vi "Autonomous Independent.vi"() -> ()   [LabVIEW 2017]
doc: "This VI is called when autonomous begins, and will automatically be terminated when autonomous ends. You can carry out timed or sensor driven robot movement independently without needing to return to the caller."
uses:
  <vilib>/Rock Robotics/WPI/ThirdParty/Sensors/navX/_TypeDefs/FRIC_navX_DeviceNumbersTypeDef.ctl
  <vilib>/Rock Robotics/WPI/Utilities/WPI_GetSetVariantRefNum.vi
  <vilib>/addons/control/pid/pid.llb/PID (DBL).vi
  <vilib>/addons/control/pid/NI_PID_pid.lvlib
  <vilib>/Rock Robotics/WPI/RobotDrive/WPI_RobotDriveArcadeDrive_Standard(NoSaturation).vi
panel:
  out "Angle 2":dbl
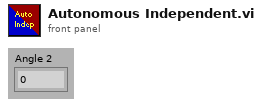
[diagram p1: front panel]
types:
  T1 = typedef "WPI_EncoderDevRef.ctl" = cluster{"DevStatus":errorcluster, "EncoderIndex":T2, "CounterIndex":T3, "DistancePerCount":dbl, "Decoding Type":T4}
  T2 = typedef "FPGA_EncoderIdx.ctl" = enum8{"Enc 0", "Enc 1", "Enc 2", "Enc 3", "Enc 4", "Enc 5", "Enc 6", "Enc 7", "Invalid"}
  T3 = typedef "FPGA_CounterCtrSystemIndex.ctl" = enum8{"Ctr 0", "Ctr 1", "Ctr 2", "Ctr 3", "Ctr 4", "Ctr 5", "Ctr 6", "Ctr 7", "Invalid"}
  T4 = typedef "WPI_EncoderType.ctl" = enum16{"1x", "2x", "4x"}
  T5 = typedef "WPI_RobotDriveDevRef.ctl" = cluster{"DevStatus":errorcluster, "Motors[]":T6[], "Square Inputs":bool, "Max Output":dbl}
  T6 = typedef "WPI_MotorControlDeviceRef.ctl" = cluster{"DeviceStatus":errorcluster, "Type":T7, "PWM":cluster{"PWM Channel":T8, "DeadBand":T9}, "CAN":cluster{"Device Number":u8, "SetOutput VI Ref":variant, "GetOutput VI Ref":variant, "Enable VI Ref":variant, "Disable VI Ref":variant, "Data":variant}, "Invert":bool, "DIO PWM":cluster{"PWM \"Enable\" Channel":T8, "DIOChannel":T10, "PWM Rate":dbl}}
  T7 = typedef "WPI_MotorControlType.ctl" = enum16{"PWM", "CAN", "DIO PWM"}
  T8 = typedef "FPGA_DIOPWMChannel.ctl" = enum8{"PWM 0", "PWM 1", "PWM 2", "PWM 3", "PWM 4", "PWM 5", "PWM 6", "PWM 7", "PWM 8", "PWM 9", "PWM MXP 0", "PWM MXP 1", "PWM MXP 2", "PWM MXP 3", "PWM MXP 4", "PWM MXP 5", "PWM MXP 6", "PWM MXP 7", "PWM MXP 8", "PWM MXP 9", "Invalid"}
  T9 = typedef "WPI_PWMDeadband.ctl" = cluster{"Name":string, "maxPositivePwm":i32, "minPositivePwm":i32, "centerPwm":i32, "maxNegativePwm":i32, "minNegativePwm":i32, "angularRange":u16}
  T10 = typedef "FPGA_DIOChannel.ctl" = enum8{"DIO 0", "DIO 1", "DIO 2", "DIO 3", "DIO 4", "DIO 5", "DIO 6", "DIO 7", "DIO 8", "DIO 9", "DIO MXP 0", "DIO MXP 1", "DIO MXP 2", "DIO MXP 3", "DIO MXP 4", "DIO MXP 5", "DIO MXP 6", "DIO MXP 7", "DIO MXP 8", "DIO MXP 9", "DIO MXP 10", "DIO MXP 11", "DIO MXP 12", "DIO MXP 13", "DIO MXP 14", "DIO MXP 15", "SPI Port CS1", "SPI Port CS2", "SPI Port CS3", "SPI Port MISO", "SPI Port MOSI", "Invalid"}
  T11 = typedef "WPI_GyroDevRef.ctl" = cluster{"DevStatus":errorcluster, "Analog Channel":T12, "Gain (VoltsPerDegree/Second)":dbl, "Gyro Type":enum16{"Analog", "XRS450"}, "Handle":i32, "SPI Bus":T13, "Device Found":bool, "Sample Rate":dbl, "Calibrate On Open":bool, "Offset":dbl}
  T12 = typedef "FPGA_AIChannel.ctl" = enum8{"AI 0", "AI 1", "AI 2", "AI 3", "AI MXP 0", "AI MXP 1", "AI MXP 2", "AI MXP 3", "Invalid"}
  T13 = typedef "spi_bus.ctl" = enum16{"SPI On-Board, CS0", "SPI On-Board, CS1", "SPI On-Board, CS2", "SPI On-Board, CS3", "SPI MXP", "Invalid"}
  T14 = typedef "FRIC_navX_DeviceNumbersTypeDef.ctl" = enum16{"Dev0", "Dev1", "Dev2", "Dev3"}
  T15 = cluster{"proportional gain (Kc)":dbl, "integral time (Ti, min)":dbl, "derivative time (Td, min)":dbl}
  T16 = cluster{"Yaw":dbl, "Roll":dbl, "Pitch":dbl, "Heading":dbl, "Fused Heading":dbl}
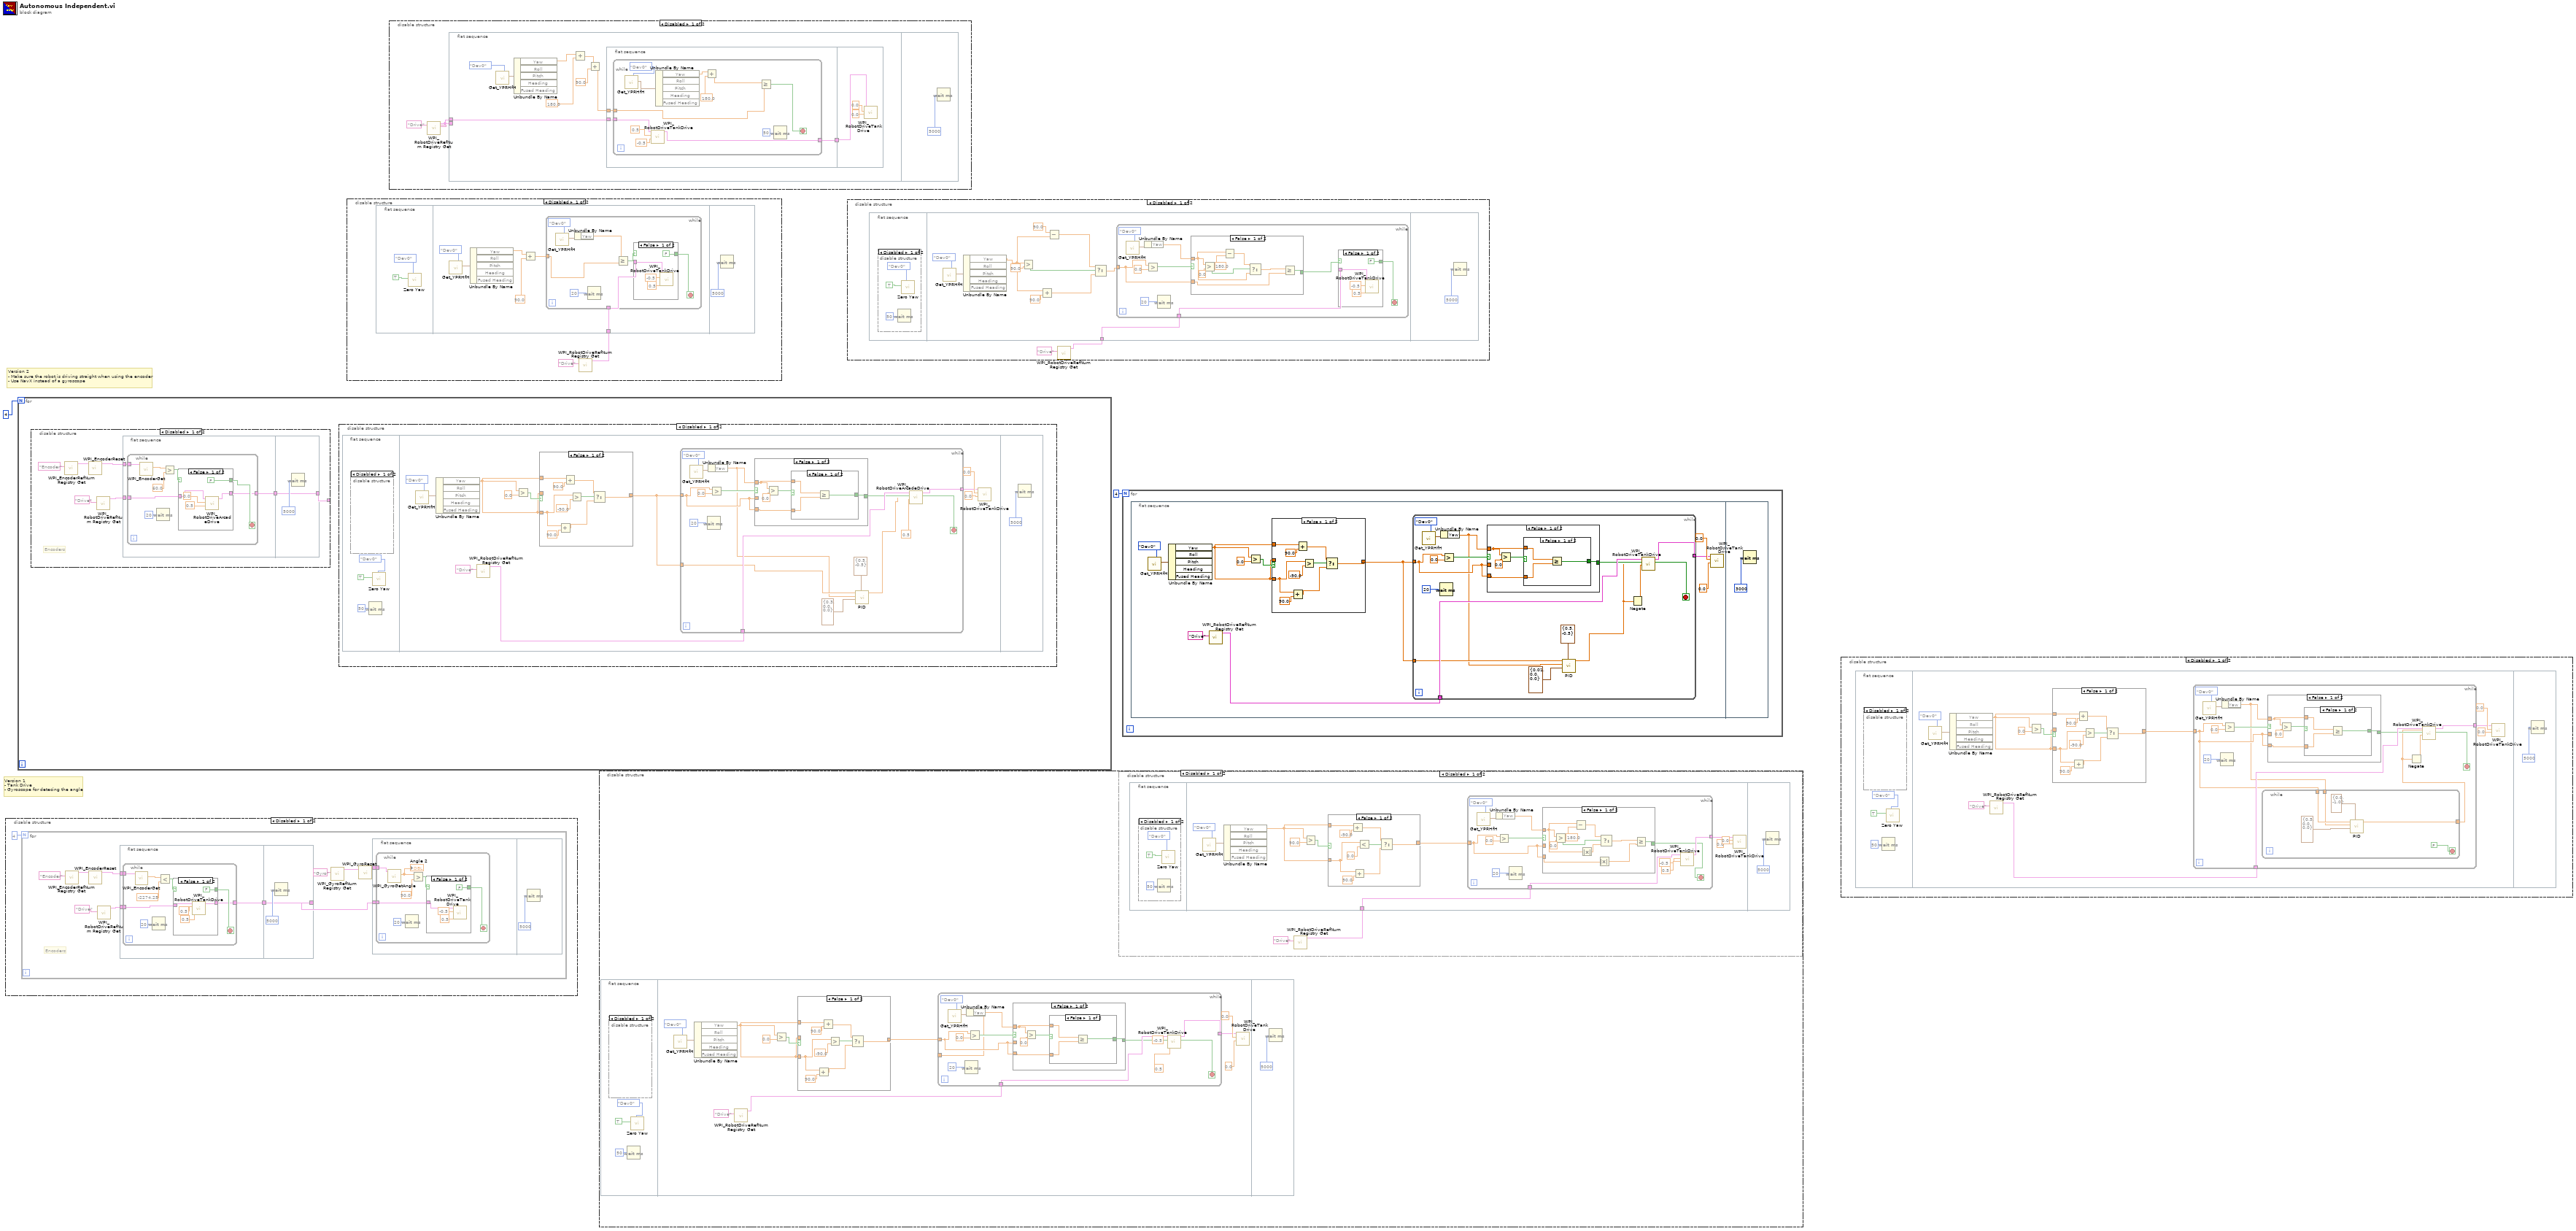
[diagram p0: block diagram]
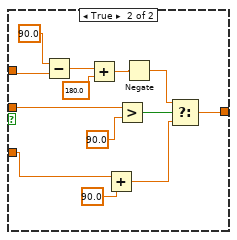
[diagram p2: hidden frame]
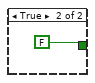
[diagram p3: hidden frame]
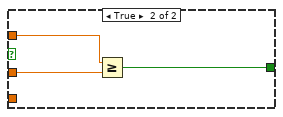
[diagram p4: hidden frame]
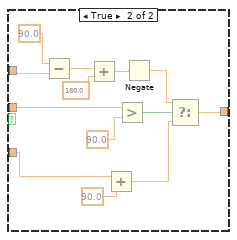
[diagram p6: hidden frame]
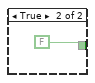
[diagram p7: hidden frame]
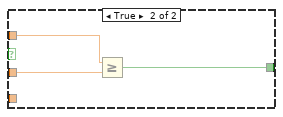
[diagram p8: hidden frame]
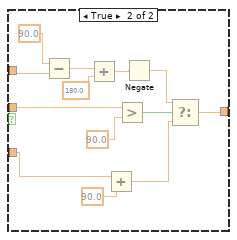
[diagram p11: hidden frame]
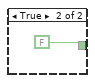
[diagram p12: hidden frame]
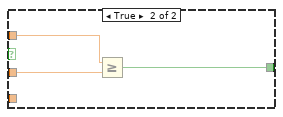
[diagram p13: hidden frame]
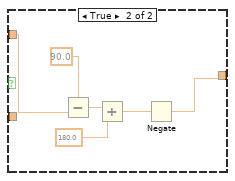
[diagram p15: hidden frame]
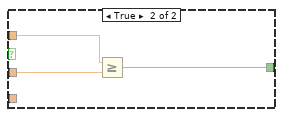
[diagram p16: hidden frame]
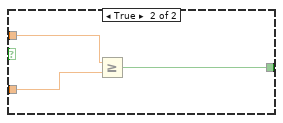
[diagram p20: hidden frame]
diagram:
  # "Version 2\n- Make sure the robot is driving straight when using the encoder\n- Use NavX instead of a gyroscope"
  # "Version 1\n- Tank Drive\n- Gyroscope for detecing the angle"
  n1 = disable-structure shown="Disabled" {
    frame Disabled {
      n2 = for {
        N: 4 -> [_]
        # "Encoders"
        n3 = call <vilib>:"WPI_EncoderRefNum Registry Get.vi"("refnum name"="Encoder") -> ("EncoderDevRef"=w10:T1)  [unwired: 9 in, 1 out]
        n4 = call <vilib>:"WPI_EncoderReset.vi"("EncoderDevRef"=w10) -> ("EncoderDevRef"=w9:T1)  [unwired: 9 in, 1 out]
        n5 = call <vilib>:"WPI_RobotDriveRefNum Registry Get.vi"("refnum name"="Drive") -> ("RobotDriveDevRef"=w13:T5)  [unwired: 9 in, 1 out]
        n6 = flat-sequence {
          tunnel: w9 -> [w34]
          tunnel: w13 -> [w33]
          tunnel: [w32] -> w4
          tunnel: [w53] -> w5
          tunnel: w4 -> [w53]
          frame #0 {
            n7 = while {
              tunnel: w34 -> [w42]
              tunnel: w33 -> [w38]
              tunnel: [w35] -> w32
              stop <- w41 stop-if-true
              n8 = call <vilib>:"WPI_EncoderGet.vi"("EncoderDevRef"=w42) -> ("Distance"=w39:dbl)  [unwired: 5 in, 5 out]
              n9 = Wait (ms)(milliseconds to wait=u32 20) -> ()  [unwired: 1 out]
              n10 = Less?(x=w39, y=-2274.25) -> (x < y?=w40:bool)
              n11 = case shown="False" w40 {
                tunnel: [FALSE TRUE] -> w41
                tunnel: w38 -> [w45 w49]
                tunnel: [w46 w48] -> w35
                frame False {
                  n12 = call <vilib>:"WPI_RobotDriveTankDrive.vi"("Right axis value"=0.5, "Left axis value"=0.5, "RobotDriveDevRef"=w45) -> ("RobotDriveDevRef"=w46:T5)  [unwired: 6 in, 2 out]
                }
                frame True {
                  n13 = call <vilib>:"WPI_RobotDriveTankDrive.vi"("Right axis value"=0.0, "Left axis value"=0.0, "RobotDriveDevRef"=w49) -> ("RobotDriveDevRef"=w48:T5)  [unwired: 6 in, 2 out]
                }
              }
            }
          }
          frame #1 {
            n14 = Wait (ms)(milliseconds to wait=u32 5000) -> ()  [unwired: 1 out]
          }
        }
        n15 = call <vilib>:"WPI_GyroRefNum Registry Get.vi"("refnum name"="Gyro") -> ("GyroDevRef"=w7:T11)  [unwired: 9 in, 1 out]
        n16 = call <vilib>:"WPI_GyroReset.vi"("GyroDevRef"=w7) -> ("GyroDevRef"=w8:T11)  [unwired: 9 in, 1 out]
        n17 = flat-sequence {
          tunnel: w8 -> [w15]
          tunnel: w5 -> [w14]
          frame #0 {
            n18 = while {
              tunnel: w15 -> [w18]
              tunnel: w14 -> [w16]
              stop <- w22 stop-if-true
              n19 = call <vilib>:"WPI_GyroGetAngle.vi"("GyroDevRef"=w18) -> ("Angle"=w17:dbl)  [unwired: 6 in, 4 out]
              "Angle 2" <- w17
              n20 = Wait (ms)(milliseconds to wait=u32 20) -> ()  [unwired: 1 out]
              n21 = Greater?(x=w17, y=90.0) -> (0:w21:bool)
              n22 = case shown="False" w21 {
                tunnel: [FALSE TRUE] -> w22
                tunnel: w16 -> [w23 w27]
                frame False {
                  n23 = call <vilib>:"WPI_RobotDriveTankDrive.vi"("Right axis value"=0.5, "Left axis value"=-0.5, "RobotDriveDevRef"=w23) -> ()  [unwired: 6 in, 3 out]
                }
                frame True {
                  n24 = call <vilib>:"WPI_RobotDriveTankDrive.vi"("Right axis value"=0.0, "Left axis value"=0.0, "RobotDriveDevRef"=w27) -> ()  [unwired: 6 in, 3 out]
                }
              }
            }
          }
          frame #1 {
            n25 = Wait (ms)(milliseconds to wait=u32 5000) -> ()  [unwired: 1 out]
          }
        }
      }
    }
    frame Enabled {
    }
  }
  n26 = for {
    N: 4 -> [_]
    n27 = disable-structure shown="Disabled" {
      disable-tunnel: [w119 _] -> _
      frame Disabled {
        # "Encoders"
        n28 = call <vilib>:"WPI_EncoderRefNum Registry Get.vi"("refnum name"="Encoder") -> ("EncoderDevRef"=w121:T1)  [unwired: 9 in, 1 out]
        n29 = call <vilib>:"WPI_EncoderReset.vi"("EncoderDevRef"=w121) -> ("EncoderDevRef"=w120:T1)  [unwired: 9 in, 1 out]
        n30 = call <vilib>:"WPI_RobotDriveRefNum Registry Get.vi"("refnum name"="Drive") -> ("RobotDriveDevRef"=w124:T5)  [unwired: 9 in, 1 out]
        n31 = flat-sequence {
          tunnel: w120 -> [w128]
          tunnel: w124 -> [w127]
          tunnel: [w126] -> w125
          tunnel: [w147] -> w119
          tunnel: w125 -> [w147]
          frame #0 {
            n32 = while {
              tunnel: w128 -> [w136]
              tunnel: w127 -> [w132]
              tunnel: [w129] -> w126
              stop <- w135 stop-if-true
              n33 = call <vilib>:"WPI_EncoderGet.vi"("EncoderDevRef"=w136) -> ("Distance"=w133:dbl)  [unwired: 5 in, 5 out]
              n34 = Wait (ms)(milliseconds to wait=u32 20) -> ()  [unwired: 1 out]
              n35 = Greater?(x=w133, y=60.0) -> (0:w134:bool)
              n36 = case shown="False" w134 {
                tunnel: [FALSE TRUE] -> w135
                tunnel: w132 -> [w139 w143]
                tunnel: [w140 w142] -> w129
                frame False {
                  n37 = call-poly <vilib>:"WPI_RobotDriveArcadeDrive.vi"("Y axis value"=0.5 ("Right axis value"), "X axis value"=0.0 ("Left axis value"), "RobotDriveDevRef"=w139) -> ("RobotDriveDevRef"=w140:T5)  [unwired: 6 in, 2 out]
                }
                frame True {
                  n38 = call <vilib>:"WPI_RobotDriveTankDrive.vi"("Right axis value"=0.0, "Left axis value"=0.0, "RobotDriveDevRef"=w143) -> ("RobotDriveDevRef"=w142:T5)  [unwired: 6 in, 2 out]
                }
              }
            }
          }
          frame #1 {
            n39 = Wait (ms)(milliseconds to wait=u32 5000) -> ()  [unwired: 1 out]
          }
        }
      }
      frame Enabled {
      }
    }
    n40 = disable-structure shown="Disabled" {
      frame Disabled {
        n41 = flat-sequence {
          frame #0 {
            n42 = disable-structure shown="Disabled" {
              frame Disabled {
              }
              frame Enabled {
              }
            }
            n43 = Wait (ms)(milliseconds to wait=u32 50) -> ()  [unwired: 1 out]
            n44 = call <vilib>:"Zero Yaw.vi"("Device Number"=FRIC_navX_DeviceNumbersTypeDef."Dev0", "Zero"=TRUE) -> ()  [unwired: 10 in]
          }
          frame #1 {
            n45 = call <vilib>:"Get_YPRHfH.vi"("Device Number"=FRIC_navX_DeviceNumbersTypeDef."Dev0") -> ("YRPHfH"=w68:T16)  [unwired: 10 in]
            n46 = Unbundle By Name(w68) -> ("Yaw"=w60:dbl)  [unwired: 4 out]
            n47 = call <vilib>:"WPI_RobotDriveRefNum Registry Get.vi"("refnum name"="Drive") -> ("RobotDriveDevRef"=w59:T5)  [unwired: 9 in, 1 out]
            n48 = Greater?(x=w60, y=0.0) -> (0:w63:bool)
            n49 = case shown="False" w63 {
              tunnel: w60 -> [w74 w82]
              tunnel: w60 -> [w71 w84]
              tunnel: [w72 w87] -> w58
              tunnel: w60 -> [_ w86]
              frame False {
                n50 = Add(x=w71, y=90.0) -> (x+y=w69:dbl)
                n51 = Add(x=w74, y=90.0) -> (x+y=w73:dbl)
                n52 = Greater?(x=w71, y=-90.0) -> (0:w76:bool)
                n53 = Select(t=w73, s=w76, f=w69) -> (s? t:f=w72:dbl)
              }
              frame True {
                n54 = Subtract(x=90.0, y=w82) -> (x-y=w81:dbl)
                n55 = Add(x=w81, y=180.0) -> (x+y=w79:dbl)
                n56 = Add(x=w84, y=90.0) -> (x+y=w88:dbl)
                n57 = Greater?(x=w86, y=90.0) -> (0:w89:bool)
                n58 = Negate(x=w79) -> (-x=w78:dbl)
                n59 = Select(t=w78, s=w89, f=w88) -> (s? t:f=w87:dbl)
              }
            }
            n60 = while {
              tunnel: w59 -> [w102]
              tunnel: [w99] -> w64
              tunnel: w58 -> [w97]
              tunnel: w58 -> [w96]
              stop <- w98 stop-if-true
              n61 = call <vilib>:"Get_YPRHfH.vi"("Device Number"=FRIC_navX_DeviceNumbersTypeDef."Dev0") -> ("YRPHfH"=w104:T16)  [unwired: 10 in]
              n62 = Wait (ms)(milliseconds to wait=u32 20) -> ()  [unwired: 1 out]
              n63 = Unbundle By Name(w104) -> ("Yaw"=w95:dbl)
              n64 = Greater?(x=w97, y=0.0) -> (0:w100:bool)
              n65 = case shown="False" w100 {
                tunnel: w95 -> [w108 w117]
                tunnel: [w106 w116] -> w98
                tunnel: w97 -> [_ w115]
                tunnel: w97 -> [w107 _]
                frame False {
                  n66 = Greater?(x=w108, y=0.0) -> (0:w109:bool)
                  n67 = case shown="False" w109 {
                    tunnel: w108 -> [w113 _]
                    tunnel: w107 -> [w112 _]
                    tunnel: [w111 FALSE] -> w106
                    frame False {
                      n68 = Greater Or Equal?(x=w113, y=w112) -> (x >= y?=w111:bool)
                    }
                    frame True {
                    }
                  }
                }
                frame True {
                  n69 = Greater Or Equal?(x=w117, y=w115) -> (x >= y?=w116:bool)
                }
              }
              n70 = call-poly <vilib>:"PID.vi"("output range"=cluster{"output high":dbl, "output low":dbl} {"output high"=0.5, "output low"=-0.5}, "PID gains"=T15 {"proportional gain (Kc)"=0.3, "integral time (Ti, min)"=0.0, "derivative time (Td, min)"=0.0}, "process variable"=w95, "setpoint"=w96) -> ("output"=w92:dbl)  [unwired: 6 in, 1 out]
              n71 = call-poly <vilib>:"WPI_RobotDriveArcadeDrive.vi"("Y axis value"=0.5, "X axis value"=w92, "RobotDriveDevRef"=w102) -> ("RobotDriveDevRef"=w99:T5)  [unwired: 6 in, 2 out]
            }
            n72 = call <vilib>:"WPI_RobotDriveTankDrive.vi"("Right axis value"=0.0, "Left axis value"=0.0, "RobotDriveDevRef"=w64) -> ()  [unwired: 6 in, 3 out]
          }
          frame #2 {
            n73 = Wait (ms)(milliseconds to wait=u32 5000) -> ()  [unwired: 1 out]
          }
        }
      }
      frame Enabled {
      }
    }
  }
  n74 = disable-structure shown="Disabled" {
    frame Disabled {
      n75 = flat-sequence {
        tunnel: w150 -> [w153]
        frame #0 {
          n76 = call <vilib>:"Zero Yaw.vi"("Device Number"=FRIC_navX_DeviceNumbersTypeDef."Dev0", "Zero"=TRUE) -> ()  [unwired: 10 in]
        }
        frame #1 {
          n77 = call <vilib>:"Get_YPRHfH.vi"("Device Number"=FRIC_navX_DeviceNumbersTypeDef."Dev0") -> ("YRPHfH"=w158:T16)  [unwired: 10 in]
          n78 = Unbundle By Name(w158) -> ("Yaw"=w156:dbl)  [unwired: 4 out]
          n79 = Add(x=w156, y=90.0) -> (x+y=w155:dbl)
          n80 = while {
            tunnel: w155 -> [w163]
            tunnel: w153 -> [w160]
            stop <- w166 stop-if-true
            n81 = call <vilib>:"Get_YPRHfH.vi"("Device Number"=FRIC_navX_DeviceNumbersTypeDef."Dev0") -> ("YRPHfH"=w162:T16)  [unwired: 10 in]
            n82 = Unbundle By Name(w162) -> ("Yaw"=w159:dbl)
            n83 = Wait (ms)(milliseconds to wait=u32 20) -> ()  [unwired: 1 out]
            n84 = Greater Or Equal?(x=w159, y=w163) -> (x >= y?=w165:bool)
            n85 = case shown="False" w165 {
              tunnel: [FALSE TRUE] -> w166
              tunnel: w160 -> [w167 w171]
              frame False {
                n86 = call <vilib>:"WPI_RobotDriveTankDrive.vi"("Right axis value"=0.5, "Left axis value"=-0.5, "RobotDriveDevRef"=w167) -> ()  [unwired: 6 in, 3 out]
              }
              frame True {
                n87 = call <vilib>:"WPI_RobotDriveTankDrive.vi"("Right axis value"=0.0, "Left axis value"=0.0, "RobotDriveDevRef"=w171) -> ()  [unwired: 6 in, 3 out]
              }
            }
          }
        }
        frame #2 {
          n88 = Wait (ms)(milliseconds to wait=u32 5000) -> ()  [unwired: 1 out]
        }
      }
      n89 = call <vilib>:"WPI_RobotDriveRefNum Registry Get.vi"("refnum name"="Drive") -> ("RobotDriveDevRef"=w150:T5)  [unwired: 9 in, 1 out]
    }
    frame Enabled {
    }
  }
  n90 = disable-structure shown="Disabled" {
    frame Disabled {
      n91 = call <vilib>:"WPI_RobotDriveRefNum Registry Get.vi"("refnum name"="Drive") -> ("RobotDriveDevRef"=w177:T5)  [unwired: 9 in, 1 out]
      n92 = flat-sequence {
        tunnel: w177 -> [_]
        tunnel: w177 -> [w182]
        frame #0 {
          n93 = call <vilib>:"Get_YPRHfH.vi"("Device Number"=FRIC_navX_DeviceNumbersTypeDef."Dev0") -> ("YRPHfH"=w186:T16)  [unwired: 10 in]
          n94 = Unbundle By Name(w186) -> ("Yaw"=w179:dbl)  [unwired: 4 out]
          n95 = Add(x=w179, y=180.0) -> (x+y=w180:dbl)
          n96 = Add(x=w180, y=90.0) -> (x+y=w185:dbl)
          n97 = flat-sequence {
            tunnel: w185 -> [w189]
            tunnel: [w188] -> w183
            tunnel: w182 -> [w187]
            tunnel: w183 -> [w202]
            frame #0 {
              n98 = while {
                tunnel: w189 -> [w199]
                tunnel: [w195] -> w188
                tunnel: w187 -> [w196]
                stop <- w198 stop-if-true
                n99 = call <vilib>:"Get_YPRHfH.vi"("Device Number"=FRIC_navX_DeviceNumbersTypeDef."Dev0") -> ("YRPHfH"=w200:T16)  [unwired: 10 in]
                n100 = call <vilib>:"WPI_RobotDriveTankDrive.vi"("Right axis value"=-0.5, "Left axis value"=0.5, "RobotDriveDevRef"=w196) -> ("RobotDriveDevRef"=w195:T5)  [unwired: 6 in, 2 out]
                n101 = Unbundle By Name(w200) -> ("Yaw"=w192:dbl)  [unwired: 4 out]
                n102 = Add(x=w192, y=180.0) -> (x+y=w190:dbl)
                n103 = Greater Or Equal?(x=w190, y=w199) -> (x >= y?=w198:bool)
                n104 = Wait (ms)(milliseconds to wait=u32 50) -> ()  [unwired: 1 out]
              }
            }
            frame #1 {
              n105 = call <vilib>:"WPI_RobotDriveTankDrive.vi"("Right axis value"=0.0, "Left axis value"=0.0, "RobotDriveDevRef"=w202) -> ()  [unwired: 6 in, 3 out]
            }
          }
        }
        frame #1 {
          n106 = Wait (ms)(milliseconds to wait=u32 5000) -> ()  [unwired: 1 out]
        }
      }
    }
    frame Enabled {
    }
  }
  n107 = disable-structure shown="Disabled" {
    frame Disabled {
      n108 = flat-sequence {
        frame #0 {
          n109 = disable-structure shown="Disabled" {
            frame Disabled {
            }
            frame Enabled {
            }
          }
          n110 = Wait (ms)(milliseconds to wait=u32 50) -> ()  [unwired: 1 out]
          n111 = call <vilib>:"Zero Yaw.vi"("Device Number"=FRIC_navX_DeviceNumbersTypeDef."Dev0", "Zero"=TRUE) -> ()  [unwired: 10 in]
        }
        frame #1 {
          n112 = call <vilib>:"Get_YPRHfH.vi"("Device Number"=FRIC_navX_DeviceNumbersTypeDef."Dev0") -> ("YRPHfH"=w219:T16)  [unwired: 10 in]
          n113 = Unbundle By Name(w219) -> ("Yaw"=w209:dbl)  [unwired: 4 out]
          n114 = call <vilib>:"WPI_RobotDriveRefNum Registry Get.vi"("refnum name"="Drive") -> ("RobotDriveDevRef"=w210:T5)  [unwired: 9 in, 1 out]
          n115 = Greater?(x=w209, y=0.0) -> (0:w214:bool)
          n116 = case shown="False" w214 {
            tunnel: w209 -> [w225 w233]
            tunnel: w209 -> [w222 w235]
            tunnel: [w223 w238] -> w212
            tunnel: w209 -> [_ w237]
            frame False {
              n117 = Add(x=w222, y=90.0) -> (x+y=w220:dbl)
              n118 = Add(x=w225, y=90.0) -> (x+y=w224:dbl)
              n119 = Greater?(x=w222, y=-90.0) -> (0:w227:bool)
              n120 = Select(t=w224, s=w227, f=w220) -> (s? t:f=w223:dbl)
            }
            frame True {
              n121 = Subtract(x=90.0, y=w233) -> (x-y=w232:dbl)
              n122 = Add(x=w232, y=180.0) -> (x+y=w230:dbl)
              n123 = Add(x=w235, y=90.0) -> (x+y=w239:dbl)
              n124 = Greater?(x=w237, y=90.0) -> (0:w240:bool)
              n125 = Negate(x=w230) -> (-x=w229:dbl)
              n126 = Select(t=w229, s=w240, f=w239) -> (s? t:f=w238:dbl)
            }
          }
          n127 = while {
            tunnel: w210 -> [w250]
            tunnel: [w246] -> w215
            tunnel: w212 -> [w245]
            tunnel: [w243] -> _
            stop <- w244 stop-if-true
            n128 = call <vilib>:"Get_YPRHfH.vi"("Device Number"=FRIC_navX_DeviceNumbersTypeDef."Dev0") -> ("YRPHfH"=w252:T16)  [unwired: 10 in]
            n129 = Wait (ms)(milliseconds to wait=u32 20) -> ()  [unwired: 1 out]
            n130 = Unbundle By Name(w252) -> ("Yaw"=w243:dbl)
            n131 = Greater?(x=w245, y=0.0) -> (0:w248:bool)
            n132 = case shown="False" w248 {
              tunnel: w243 -> [w256 w265]
              tunnel: [w254 w264] -> w244
              tunnel: w245 -> [_ w263]
              tunnel: w245 -> [w255 _]
              frame False {
                n133 = Greater?(x=w256, y=0.0) -> (0:w257:bool)
                n134 = case shown="False" w257 {
                  tunnel: w256 -> [w261 _]
                  tunnel: w255 -> [w260 _]
                  tunnel: [w259 FALSE] -> w254
                  frame False {
                    n135 = Greater Or Equal?(x=w261, y=w260) -> (x >= y?=w259:bool)
                  }
                  frame True {
                  }
                }
              }
              frame True {
                n136 = Greater Or Equal?(x=w265, y=w263) -> (x >= y?=w264:bool)
              }
            }
            n137 = call <vilib>:"WPI_RobotDriveTankDrive.vi"("Right axis value"=0.5, "Left axis value"=-0.5, "RobotDriveDevRef"=w250) -> ("RobotDriveDevRef"=w246:T5)  [unwired: 6 in, 2 out]
          }
          n138 = call <vilib>:"WPI_RobotDriveTankDrive.vi"("Right axis value"=0.0, "Left axis value"=0.0, "RobotDriveDevRef"=w215) -> ()  [unwired: 6 in, 3 out]
        }
        frame #2 {
          n139 = Wait (ms)(milliseconds to wait=u32 5000) -> ()  [unwired: 1 out]
        }
      }
      n140 = disable-structure shown="Disabled" {
        frame Disabled {
          n141 = flat-sequence {
            tunnel: w268 -> [w279]
            frame #0 {
              n142 = disable-structure shown="Disabled" {
                frame Disabled {
                  n143 = Wait (ms)(milliseconds to wait=u32 50) -> ()  [unwired: 1 out]
                  n144 = call <vilib>:"Zero Yaw.vi"("Device Number"=FRIC_navX_DeviceNumbersTypeDef."Dev0", "Zero"=TRUE) -> ()  [unwired: 10 in]
                }
                frame Enabled {
                }
              }
            }
            frame #1 {
              n145 = call <vilib>:"Get_YPRHfH.vi"("Device Number"=FRIC_navX_DeviceNumbersTypeDef."Dev0") -> ("YRPHfH"=w281:T16)  [unwired: 10 in]
              n146 = Unbundle By Name(w281) -> ("Yaw"=w273:dbl)  [unwired: 4 out]
              n147 = Greater?(x=w273, y=90.0) -> (0:w275:bool)
              n148 = case shown="False" w275 {
                tunnel: w273 -> [w287 w295]
                tunnel: w273 -> [w283 _]
                tunnel: [w282 w291] -> w272
                frame False {
                  n149 = Add(x=w287, y=-90.0) -> (x+y=w285:dbl)
                  n150 = Add(x=w283, y=90.0) -> (x+y=w284:dbl)
                  n151 = Less?(x=w283, y=0.0) -> (x < y?=w289:bool)
                  n152 = Select(t=w285, s=w289, f=w284) -> (s? t:f=w282:dbl)
                }
                frame True {
                  n153 = Subtract(x=90.0, y=w295) -> (x-y=w294:dbl)
                  n154 = Add(x=w294, y=180.0) -> (x+y=w292:dbl)
                  n155 = Negate(x=w292) -> (-x=w291:dbl)
                }
              }
              n156 = while {
                tunnel: w279 -> [w305]
                tunnel: [w299] -> w276
                tunnel: w272 -> [w297]
                stop <- w298 stop-if-true
                n157 = call <vilib>:"Get_YPRHfH.vi"("Device Number"=FRIC_navX_DeviceNumbersTypeDef."Dev0") -> ("YRPHfH"=w307:T16)  [unwired: 10 in]
                n158 = Unbundle By Name(w307) -> ("Yaw"=w302:dbl)
                n159 = Greater?(x=w297, y=0.0) -> (0:w303:bool)
                n160 = Wait (ms)(milliseconds to wait=u32 20) -> ()  [unwired: 1 out]
                n161 = case shown="False" w303 {
                  tunnel: w302 -> [w309 w321]
                  tunnel: [w316 w320] -> w298
                  tunnel: w297 -> [_ w319]
                  tunnel: w297 -> [w312 _]
                  frame False {
                    n162 = Greater?(x=w309, y=0.0) -> (0:w317:bool)
                    n163 = Subtract(x=w309, y=180.0) -> (x-y=w315:dbl)
                    n164 = Absolute Value(x=w309) -> (abs(x)=w310:dbl)
                    n165 = Absolute Value(x=w312) -> (abs(x)=w311:dbl)
                    n166 = Select(t=w315, s=w317, f=w310) -> (s? t:f=w314:dbl)
                    n167 = Greater Or Equal?(x=w314, y=w311) -> (x >= y?=w316:bool)
                  }
                  frame True {
                    n168 = Greater Or Equal?(x=w321, y=w319) -> (x >= y?=w320:bool)
                  }
                }
                n169 = call <vilib>:"WPI_RobotDriveTankDrive.vi"("Right axis value"=0.5, "Left axis value"=-0.5, "RobotDriveDevRef"=w305) -> ("RobotDriveDevRef"=w299:T5)  [unwired: 6 in, 2 out]
              }
              n170 = call <vilib>:"WPI_RobotDriveTankDrive.vi"("Right axis value"=0.0, "Left axis value"=0.0, "RobotDriveDevRef"=w276) -> ()  [unwired: 6 in, 3 out]
            }
            frame #2 {
              n171 = Wait (ms)(milliseconds to wait=u32 5000) -> ()  [unwired: 1 out]
            }
          }
          n172 = call <vilib>:"WPI_RobotDriveRefNum Registry Get.vi"("refnum name"="Drive") -> ("RobotDriveDevRef"=w268:T5)  [unwired: 9 in, 1 out]
        }
        frame Enabled {
        }
      }
    }
    frame Enabled {
    }
  }
  n173 = disable-structure shown="Disabled" {
    frame Disabled {
      n174 = flat-sequence {
        tunnel: w323 -> [w336]
        frame #0 {
          n175 = disable-structure shown="Disabled" {
            frame Disabled {
              n176 = Wait (ms)(milliseconds to wait=u32 50) -> ()  [unwired: 1 out]
              n177 = call <vilib>:"Zero Yaw.vi"("Device Number"=FRIC_navX_DeviceNumbersTypeDef."Dev0", "Zero"=TRUE) -> ()  [unwired: 10 in]
            }
            frame Enabled {
            }
          }
        }
        frame #1 {
          n178 = call <vilib>:"Get_YPRHfH.vi"("Device Number"=FRIC_navX_DeviceNumbersTypeDef."Dev0") -> ("YRPHfH"=w338:T16)  [unwired: 10 in]
          n179 = Unbundle By Name(w338) -> ("Yaw"=w331:dbl)  [unwired: 4 out]
          n180 = Greater?(x=w331, y=90.0) -> (0:w334:bool)
          n181 = Add(x=w331, y=90.0) -> (x+y=w328:dbl)
          n182 = Subtract(x=90.0, y=w331) -> (x-y=w329:dbl)
          n183 = Select(t=w329, s=w334, f=w328) -> (s? t:f=w333:dbl)
          n184 = while {
            tunnel: w336 -> [w344]
            tunnel: w333 -> [w341]
            stop <- w348 stop-if-true
            n185 = call <vilib>:"Get_YPRHfH.vi"("Device Number"=FRIC_navX_DeviceNumbersTypeDef."Dev0") -> ("YRPHfH"=w346:T16)  [unwired: 10 in]
            n186 = Unbundle By Name(w346) -> ("Yaw"=w340:dbl)
            n187 = Greater?(x=w341, y=0.0) -> (0:w342:bool)
            n188 = Wait (ms)(milliseconds to wait=u32 20) -> ()  [unwired: 1 out]
            n189 = case shown="False" w342 {
              tunnel: w341 -> [w354 w359]
              tunnel: w340 -> [w349 w358]
              tunnel: [w353 w357] -> w339
              frame False {
                n190 = Greater?(x=w349, y=0.0) -> (0:w355:bool)
                n191 = Subtract(x=w349, y=180.0) -> (x-y=w352:dbl)
                n192 = Select(t=w352, s=w355, f=w349) -> (s? t:f=w351:dbl)
                n193 = Greater Or Equal?(x=w351, y=w354) -> (x >= y?=w353:bool)
              }
              frame True {
                n194 = Greater Or Equal?(x=w358, y=w359) -> (x >= y?=w357:bool)
              }
            }
            n195 = case shown="False" w339 {
              tunnel: [FALSE TRUE] -> w348
              tunnel: w344 -> [w360 w364]
              frame False {
                n196 = call <vilib>:"WPI_RobotDriveTankDrive.vi"("Right axis value"=0.5, "Left axis value"=-0.5, "RobotDriveDevRef"=w360) -> ()  [unwired: 6 in, 3 out]
              }
              frame True {
                n197 = call <vilib>:"WPI_RobotDriveTankDrive.vi"("Right axis value"=0.0, "Left axis value"=0.0, "RobotDriveDevRef"=w364) -> ()  [unwired: 6 in, 3 out]
              }
            }
          }
        }
        frame #2 {
          n198 = Wait (ms)(milliseconds to wait=u32 5000) -> ()  [unwired: 1 out]
        }
      }
      n199 = call <vilib>:"WPI_RobotDriveRefNum Registry Get.vi"("refnum name"="Drive") -> ("RobotDriveDevRef"=w323:T5)  [unwired: 9 in, 1 out]
    }
    frame Enabled {
    }
  }
  n200 = for {
    N: 4 -> [_]
    n201 = flat-sequence {
      frame #0 {
        n202 = call <vilib>:"Get_YPRHfH.vi"("Device Number"=FRIC_navX_DeviceNumbersTypeDef."Dev0") -> ("YRPHfH"=w379:T16)  [unwired: 10 in]
        n203 = Unbundle By Name(w379) -> ("Yaw"=w370:dbl)  [unwired: 4 out]
        n204 = call <vilib>:"WPI_RobotDriveRefNum Registry Get.vi"("refnum name"="Drive") -> ("RobotDriveDevRef"=w371:T5)  [unwired: 9 in, 1 out]
        n205 = Greater?(x=w370, y=0.0) -> (0:w374:bool)
        n206 = case shown="False" w374 {
          tunnel: w370 -> [w385 w393]
          tunnel: w370 -> [w382 w395]
          tunnel: [w383 w398] -> w369
          tunnel: w370 -> [_ w397]
          frame False {
            n207 = Add(x=w382, y=90.0) -> (x+y=w380:dbl)
            n208 = Add(x=w385, y=90.0) -> (x+y=w384:dbl)
            n209 = Greater?(x=w382, y=-90.0) -> (0:w387:bool)
            n210 = Select(t=w384, s=w387, f=w380) -> (s? t:f=w383:dbl)
          }
          frame True {
            n211 = Subtract(x=90.0, y=w393) -> (x-y=w392:dbl)
            n212 = Add(x=w392, y=180.0) -> (x+y=w390:dbl)
            n213 = Add(x=w395, y=90.0) -> (x+y=w399:dbl)
            n214 = Greater?(x=w397, y=90.0) -> (0:w400:bool)
            n215 = Negate(x=w390) -> (-x=w389:dbl)
            n216 = Select(t=w389, s=w400, f=w399) -> (s? t:f=w398:dbl)
          }
        }
        n217 = while {
          tunnel: w371 -> [w413]
          tunnel: [w410] -> w375
          tunnel: w369 -> [w409]
          tunnel: w369 -> [w403]
          stop <- w408 stop-if-true
          n218 = call <vilib>:"Get_YPRHfH.vi"("Device Number"=FRIC_navX_DeviceNumbersTypeDef."Dev0") -> ("YRPHfH"=w415:T16)  [unwired: 10 in]
          n219 = Wait (ms)(milliseconds to wait=u32 20) -> ()  [unwired: 1 out]
          n220 = Unbundle By Name(w415) -> ("Yaw"=w402:dbl)
          n221 = Greater?(x=w409, y=0.0) -> (0:w411:bool)
          n222 = case shown="False" w411 {
            tunnel: w402 -> [w419 w428]
            tunnel: [w417 w427] -> w408
            tunnel: w409 -> [_ w426]
            tunnel: w409 -> [w418 _]
            frame False {
              n223 = Greater?(x=w419, y=0.0) -> (0:w420:bool)
              n224 = case shown="False" w420 {
                tunnel: w419 -> [w424 _]
                tunnel: w418 -> [w423 _]
                tunnel: [w422 FALSE] -> w417
                frame False {
                  n225 = Greater Or Equal?(x=w424, y=w423) -> (x >= y?=w422:bool)
                }
                frame True {
                }
              }
            }
            frame True {
              n226 = Greater Or Equal?(x=w428, y=w426) -> (x >= y?=w427:bool)
            }
          }
          n227 = call-poly <vilib>:"PID.vi"("output range"=cluster{"output high":dbl, "output low":dbl} {"output high"=0.5, "output low"=-0.5}, "PID gains"=T15 {"proportional gain (Kc)"=0.01, "integral time (Ti, min)"=0.0, "derivative time (Td, min)"=0.0}, "process variable"=w402, "setpoint"=w403) -> ("output"=w405:dbl)  [unwired: 6 in, 1 out]
          n228 = Negate(x=w405) -> (-x=w404:dbl)
          n229 = call <vilib>:"WPI_RobotDriveTankDrive.vi"("Right axis value"=w404, "Left axis value"=w405, "RobotDriveDevRef"=w413) -> ("RobotDriveDevRef"=w410:T5)  [unwired: 6 in, 2 out]
        }
        n230 = call <vilib>:"WPI_RobotDriveTankDrive.vi"("Right axis value"=0.0, "Left axis value"=0.0, "RobotDriveDevRef"=w375) -> ()  [unwired: 6 in, 3 out]
      }
      frame #1 {
        n231 = Wait (ms)(milliseconds to wait=u32 3000) -> ()  [unwired: 1 out]
      }
    }
  }
  n232 = disable-structure shown="Disabled" {
    frame Disabled {
      n233 = flat-sequence {
        frame #0 {
          n234 = disable-structure shown="Disabled" {
            frame Disabled {
            }
            frame Enabled {
            }
          }
          n235 = Wait (ms)(milliseconds to wait=u32 50) -> ()  [unwired: 1 out]
          n236 = call <vilib>:"Zero Yaw.vi"("Device Number"=FRIC_navX_DeviceNumbersTypeDef."Dev0", "Zero"=TRUE) -> ()  [unwired: 10 in]
        }
        frame #1 {
          n237 = call <vilib>:"Get_YPRHfH.vi"("Device Number"=FRIC_navX_DeviceNumbersTypeDef."Dev0") -> ("YRPHfH"=w443:T16)  [unwired: 10 in]
          n238 = Unbundle By Name(w443) -> ("Yaw"=w435:dbl)  [unwired: 4 out]
          n239 = call <vilib>:"WPI_RobotDriveRefNum Registry Get.vi"("refnum name"="Drive") -> ("RobotDriveDevRef"=w433:T5)  [unwired: 9 in, 1 out]
          n240 = Greater?(x=w435, y=0.0) -> (0:w438:bool)
          n241 = case shown="False" w438 {
            tunnel: w435 -> [w449 w457]
            tunnel: w435 -> [w446 w459]
            tunnel: [w447 w462] -> w434
            tunnel: w435 -> [_ w461]
            frame False {
              n242 = Add(x=w446, y=90.0) -> (x+y=w444:dbl)
              n243 = Add(x=w449, y=90.0) -> (x+y=w448:dbl)
              n244 = Greater?(x=w446, y=-90.0) -> (0:w451:bool)
              n245 = Select(t=w448, s=w451, f=w444) -> (s? t:f=w447:dbl)
            }
            frame True {
              n246 = Subtract(x=90.0, y=w457) -> (x-y=w456:dbl)
              n247 = Add(x=w456, y=180.0) -> (x+y=w454:dbl)
              n248 = Add(x=w459, y=90.0) -> (x+y=w463:dbl)
              n249 = Greater?(x=w461, y=90.0) -> (0:w464:bool)
              n250 = Negate(x=w454) -> (-x=w453:dbl)
              n251 = Select(t=w453, s=w464, f=w463) -> (s? t:f=w462:dbl)
            }
          }
          n252 = while {
            tunnel: w433 -> [w474]
            tunnel: [w471] -> w439
            tunnel: w434 -> [w469]
            stop <- w470 stop-if-true
            n253 = call <vilib>:"Get_YPRHfH.vi"("Device Number"=FRIC_navX_DeviceNumbersTypeDef."Dev0") -> ("YRPHfH"=w476:T16)  [unwired: 10 in]
            n254 = Wait (ms)(milliseconds to wait=u32 20) -> ()  [unwired: 1 out]
            n255 = Unbundle By Name(w476) -> ("Yaw"=w468:dbl)
            n256 = Greater?(x=w469, y=0.0) -> (0:w472:bool)
            n257 = while {
              tunnel: [w481] -> w467
              tunnel: w469 -> [w479]
              tunnel: w468 -> [w478]
              stop <- FALSE stop-if-true
              n258 = call-poly <vilib>:"PID.vi"("output range"=cluster{"output high":dbl, "output low":dbl} {"output high"=0.0, "output low"=-1.0}, "PID gains"=T15 {"proportional gain (Kc)"=0.5, "integral time (Ti, min)"=0.0, "derivative time (Td, min)"=0.0}, "process variable"=w478, "setpoint"=w479) -> ("output"=w481:dbl)  [unwired: 6 in, 1 out]
            }
            n259 = case shown="False" w472 {
              tunnel: w468 -> [w486 w495]
              tunnel: [w484 w494] -> w470
              tunnel: w469 -> [_ w493]
              tunnel: w469 -> [w485 _]
              frame False {
                n260 = Greater?(x=w486, y=0.0) -> (0:w487:bool)
                n261 = case shown="False" w487 {
                  tunnel: w486 -> [w491 _]
                  tunnel: w485 -> [w490 _]
                  tunnel: [w489 FALSE] -> w484
                  frame False {
                    n262 = Greater Or Equal?(x=w491, y=w490) -> (x >= y?=w489:bool)
                  }
                  frame True {
                  }
                }
              }
              frame True {
                n263 = Greater Or Equal?(x=w495, y=w493) -> (x >= y?=w494:bool)
              }
            }
            n264 = Negate(x=w467) -> (-x=w466:dbl)
            n265 = call <vilib>:"WPI_RobotDriveTankDrive.vi"("Right axis value"=w466, "Left axis value"=w467, "RobotDriveDevRef"=w474) -> ("RobotDriveDevRef"=w471:T5)  [unwired: 6 in, 2 out]
          }
          n266 = call <vilib>:"WPI_RobotDriveTankDrive.vi"("Right axis value"=0.0, "Left axis value"=0.0, "RobotDriveDevRef"=w439) -> ()  [unwired: 6 in, 3 out]
        }
        frame #2 {
          n267 = Wait (ms)(milliseconds to wait=u32 5000) -> ()  [unwired: 1 out]
        }
      }
    }
    frame Enabled {
    }
  }
